vi "tele.vi"() -> ()   [LabVIEW 2012, in "BlockParty4150.lvrbt"]
uses:
  BlockParty4150.lvrbt
  <vilib>/NXT/Hardware/Plugins/Tetrix DC Motor/TetrixDCMotorAddress.ctl
  <vilib>/FTC/FTC Calculate Drive Power - Tank.vi
  <vilib>/NXT/NXTIO Xnodes/NXTIONodeSubVIs/TETRIX IO Move DC Motors.vi
  <vilib>/NXT/NXTIO Xnodes/NXTIONodeSubVIs/TETRIX IO Check Battery.vi
  <vilib>/NXT/NXTIO Xnodes/NXTIONodeSubVIs/TETRIX IO Stop DC Motors.vi
  <vilib>/NXT/NXTIO Xnodes/AddressXNode/NXTIOAddress.xnode
  <vilib>/NXT/Subs/LVHSConnector.ctl
  <vilib>/NXT/NXTIO Xnodes/NXTIOXNode/NXTIO.xnode
  <vilib>/NXT/LegoClasses/BrickReference/BrickReference.lvclass
panel:
  out "Enabled?":enum16{"Disabled", "Enabled"}(ring)
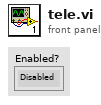
[diagram p1: front panel]
types:
  T1 = typedef "LVHSConnector.ctl" = refnum<class "BrickReference.lvclass">
  T2 = typedef "TetrixDCMotorAddress.ctl" = i16
  T3 = cluster{"TetrixDCMotor":T2, "TetrixDCMotor 2":T2}
  T4 = typedef "FTC ControllerState.ctl" = cluster{"Left X":i8, "Left Y":i8, "Right X":i8, "Right Y":i8, "Button Encoding 9-12":u8, "Button Encoding 1-8":u8, "POV":T5}
  T5 = typedef "FTC POVState.ctl" = i8
  T6 = typedef "FTC ButtonEventType.ctl" = enum16{"Pressed", "Released"}
  T7 = cluster{"Button ID":enum16{"None", "Button 1", "Button 2", "Button 3", "Button 4", "Button 5", "Button 6", "Button 7", "Button 8", "Button 9", "Button 10", "Button 11", "Button 12", "POV Up", "POV Up Right", "POV Right", "POV Down Right", "POV Down", "POV Down Left", "POV Left", "POV Up Left"}, "Event Type":T6}[]
  T8 = enum16{"None", "Button 1", "Button 2", "Button 3", "Button 4", "Button 5", "Button 6", "Button 7", "Button 8", "Button 9", "Button 10", "Button 11", "Button 12", "POV Up", "POV Up Right", "POV Right", "POV Down Right", "POV Down", "POV Down Left", "POV Left", "POV Up Left"}
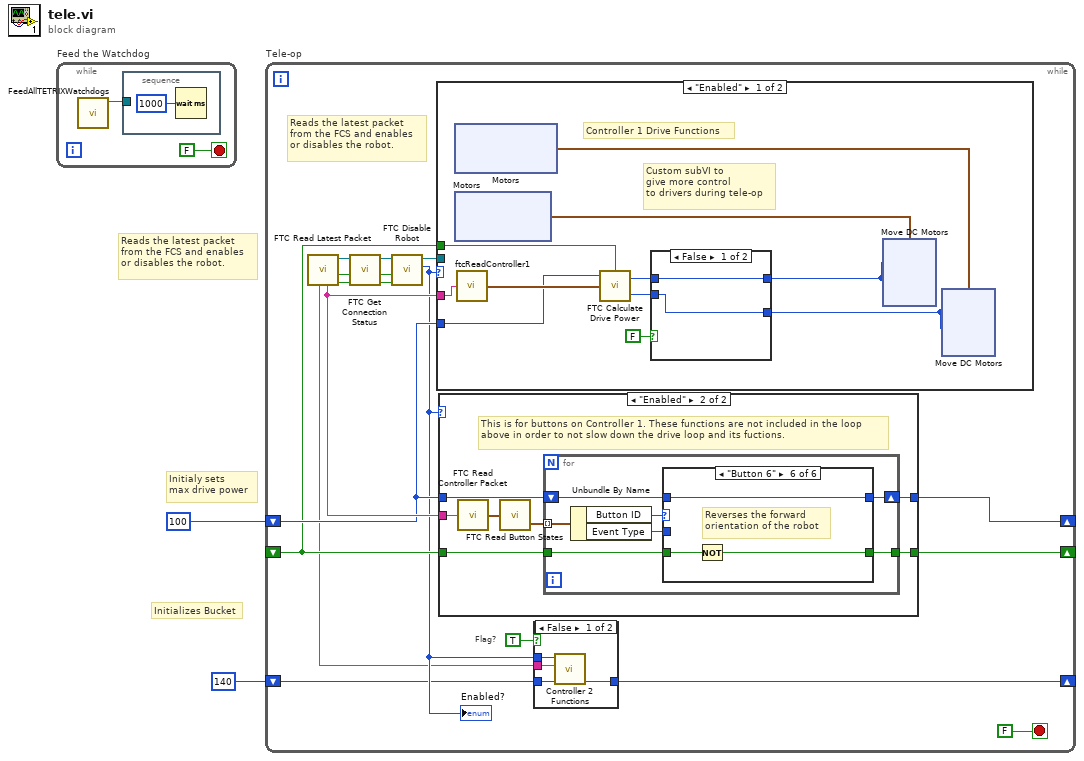
[diagram p0: block diagram]
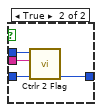
[diagram p2: hidden frame]
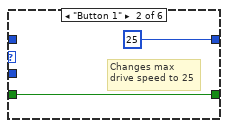
[diagram p5: hidden frame]
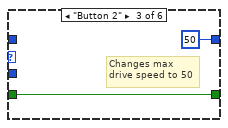
[diagram p6: hidden frame]
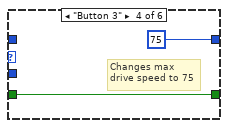
[diagram p7: hidden frame]
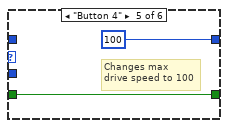
[diagram p8: hidden frame]
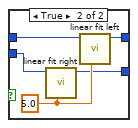
[diagram p9: hidden frame]
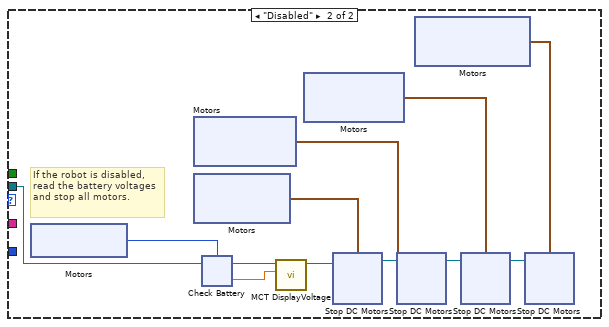
[diagram p10: hidden frame]
diagram:
  # "Initializes Bucket"
  # "Initialy sets\nmax drive power"
  # "Reads the latest packet\nfrom the FCS and enables\nor disables the robot."
  n1 = while "Feed the Watchdog" {
    stop <- FALSE stop-if-true
    n2 = call <vilib>:"FeedAllTETRIXWatchdogs.vi"() -> ("NXT"=w3:T1)  [unwired: 11 in]
    n3 = stacked-sequence {
      tunnel: w3 -> [_]
      frame #0 {
        n4 = Wait (ms)(milliseconds to wait=u32 1000) -> ()  [unwired: 1 out]
      }
    }
  }
  n5 = while "Tele-op" {
    shift-right: [w15] -> _
    shift-left: i8 100 ("Power Level (50)") -> [w12]
    shift-right: [w14] -> _
    shift-left: _ -> [w11]
    shift-right: [w6] -> _
    shift-left: u8 140 ("AutoArmIn") -> [w8]
    stop <- FALSE stop-if-true
    # "Flag?"
    # "Reads the latest packet\nfrom the FCS and enables\nor disables the robot."
    n6 = call <vilib>:"FTC Read Latest Packet.vi"() -> ("Packet Received?"=w22:bool, "Stopped?"=w20:bool, "NXT"=w21:T1, "Controller 1"=w13:string, "Controller 2"=w9:string)  [unwired: 6 in, 1 out]
    n7 = call <vilib>:"FTC Get Connection Status.vi"("Packet Received?"=w22, "Stopped?"=w20, "NXT"=w21) -> ("Online?"=w17:bool, "Stopped?"=w18:bool, "NXT"=w19:T1)  [unwired: 5 in]
    n8 = call <vilib>:"FTC Disable Robot.vi"("Online?"=w17, "Stopped?"=w18, "NXT"=w19) -> ("Enabled?"=w10:enum16{"Disabled", "Enabled"}, "NXT"=w16:T1)  [unwired: 3 in]
    "Enabled?" <- w10
    n9 = case "disableCase" shown="\"Enabled\"" w10 {
      tunnel: w13 -> [w71 _]
      tunnel: w16 -> [_ w112]
      tunnel: w12 -> [w67 _]
      tunnel: w11 -> [w66 _]
      frame "Enabled" {
        # "Controller 1 Drive Functions"
        # "Custom subVI to\ngive more control\nto drivers during tele-op"
        n10 = xnode ("Motors")() -> ("Motor"=w69:cluster{"TetrixDCMotor":T2, "TetrixDCMotor":T2})
        n11 = xnode ("Motors")() -> ("Motor"=w68:cluster{"TetrixDCMotor":T2, "TetrixDCMotor":T2})
        n12 = call "ftcReadController1"("Packet"=w71) -> ("Controller State"=w70:T4)  [unwired: 4 in]
        n13 = call-poly <vilib>:"FTC Calculate Drive Power.vi"("Reverse"=w66, "Controller State"=w70, "Power Level (50)"=w67) -> ("Right Motor Power"=w64:i8, "Left Motor Power"=w65:i8)  [unwired: 1 in]
        n14 = case shown="False" FALSE {
          tunnel: w65 -> [w73 w78]
          tunnel: [w73 w77] -> w62
          tunnel: w64 -> [w72 w76]
          tunnel: [w72 w74] -> w61
          frame False {
          }
          frame True {
            w75 = 5.0 ("# of samples")
            n15 = call "linear fit right.vi"("# of samples"=w75, "Left in"=w76) -> ("Left out"=w74:i8)  [unwired: 9 in]
            n16 = call "linear fit left.vi"("# of samples"=w75, "Left in"=w78) -> ("Left out"=w77:i8)  [unwired: 9 in]
          }
        }
        n17 = xnode ("Move DC Motors")("Power/Speed 2"=w62, "Power/Speed 1"=w62, "Motors"=w68) -> ()  [unwired: 1 in, 1 out]
        n18 = xnode ("Move DC Motors")("Power/Speed 2"=w61, "Power/Speed 1"=w61, "Motors"=w69) -> ()  [unwired: 1 in, 1 out]
      }
      frame "Disabled" {
        # "If the robot is disabled, read the battery voltages and stop all motors."
        n19 = xnode ("Motors")() -> ("Motor"=w111:T2)
        n20 = xnode "Motors"() -> ("Motor"=w106:cluster{"TetrixDCMotor":T2, "TetrixDCMotor":T2})
        n21 = xnode "Motors"() -> ("Motor"=w108:cluster{"TetrixDCMotor":T2, "TetrixDCMotor":T2})
        n22 = xnode ("Check Battery")("Motors"=w111, "NXT"=w112) -> ("Voltage 1"=w110:sgl, "NXT"=w109:T1)
        n23 = call <vilib>:"MCT DisplayVoltage.vi"("Motor Voltage"=w110, "NXT"=w109) -> ("NXT"=w107:T1)  [unwired: 9 in]
        n24 = xnode "Motors"() -> ("Motor"=w104:cluster{"TetrixDCMotor":T2, "TetrixDCMotor":T2})
        n25 = xnode "Stop DC Motors"("Motors"=w108, "NXT"=w107) -> ("NXT"=w105:T1)
        n26 = xnode "Stop DC Motors"("Motors"=w106, "NXT"=w105) -> ("NXT"=w103:T1)
        n27 = xnode "Motors"() -> ("Motor"=w102:cluster{"TetrixDCMotor":T2, "TetrixDCMotor":T2})
        n28 = xnode "Stop DC Motors"("Motors"=w104, "NXT"=w103) -> ("NXT"=w101:T1)
        n29 = xnode "Stop DC Motors"("Motors"=w102, "NXT"=w101) -> ()  [unwired: 1 out]
      }
    }
    n30 = case shown="\"Enabled\"" w10 {
      tunnel: w13 -> [_ w40]
      tunnel: [w33 w37] -> w15
      tunnel: w12 -> [w33 w36]
      tunnel: [w32 w35] -> w14
      tunnel: w11 -> [w32 w34]
      frame "Disabled", Default {
      }
      frame "Enabled" {
        # "This is for buttons on Controller 1. These functions are not included in the loop above in order to not slow down the drive loop and its fuctions."
        n31 = call <vilib>:"FTC Read Controller Packet.vi"("Packet"=w40) -> ("Controller State"=w39:T4)  [unwired: 4 in]
        n32 = call <vilib>:"FTC Read Button States.vi"("Controller State"=w39) -> ("Button Events"=w38:T7)  [unwired: 2 in, 1 out]
        n33 = for {
          tunnel: w38 -> [w47] mode=indexing
          tunnel: [w42] -> w35
          tunnel: w34 -> [w41]
          shift-right: [w44] -> w37
          shift-left: w36 -> [w43]
          n34 = Unbundle By Name(w47) -> ("Button ID"=w46:T8, "Event Type"=w45:T6)
          n35 = case shown="\"Button 6\"" w46 {
            tunnel: w45 -> [_ _ _ _ _ _]
            tunnel: [w49 i8 25 ("Power Level (50)") i8 50 ("Power Level (50)") i8 75 ("Power Level (50)") i8 100 ("Power Level (50)") w60] -> w44
            tunnel: w43 -> [w49 _ _ _ _ w60]
            tunnel: [w48 w50 w52 w54 w56 w59] -> w42
            tunnel: w41 -> [w48 w50 w52 w54 w56 w58]
            frame "None", Default {
            }
            frame "Button 1" {
              # "Changes max\ndrive speed to 25"
            }
            frame "Button 2" {
              # "Changes max\ndrive speed to 50"
            }
            frame "Button 3" {
              # "Changes max\ndrive speed to 75"
            }
            frame "Button 4" {
              # "Changes max\ndrive speed to 100"
            }
            frame "Button 6" {
              # "Reverses the forward\norientation of the robot"
              n36 = Not(x=w58) -> (.not. x?=w59:bool)
            }
          }
        }
      }
    }
    n37 = case shown="False" TRUE {
      tunnel: w10 -> [w27 w31]
      tunnel: w9 -> [w26 w30]
      tunnel: w8 -> [w25 w29]
      tunnel: [w24 w28] -> w6
      frame False {
        n38 = call "Controller 2 Functions.vi"("AutoArmIn"=w25, "Controller in"=w26, "Enabled?"=w27) -> ("AutoArm Out"=w24:u8)  [unwired: 8 in]
      }
      frame True {
        n39 = call "Ctrlr 2 Flag.vi"("AutoArmIn"=w29, "Controller in"=w30, "Enabled?"=w31) -> ("AutoArm Out"=w28:u8)  [unwired: 8 in]
      }
    }
  }
